vi "robot_state_machine1.vi"() -> ()   [LabVIEW 2015]
panel:
  out "angle error":dbl
  out "orientation theta desired":dbl
  out "start y":dbl
  out "start x 2":dbl=1.0
  out "x traveled 2":dbl
  out "y traveled 2":dbl
  out "avg 124":dbl
  out "avg 457":dbl
  out "psi dot 2":dbl
  out "distance traveled 2":dbl
  out "y dot 2":dbl
  out "x dot 2":dbl
  out "x position 2":dbl
  out "y position 2":dbl
  out "reset x y 2":dbl
  out "Tick Count(mSec) 2":u32 caption="Tick Count(mSec)"
  out "right":dbl
  out "left":dbl
  in  "x goal":dbl=10.0
  out "goal reached":bool=TRUE
  out "scale":dbl=1.0
  out "x/y":dbl
  out "stop switch":dbl=1.0
  in  "Encoder Reset":bool
  out "ENC.B_c.CNTR":i32
  out "ENC.B_b.CNTR":i32
  out "ENC.B_a.CNTR":i32
  out "ENC.A_c.CNTR":i32
  out "ENC.A_b.CNTR":i32
  out "ENC.A_a.CNTR":i32
  out "slope desired":dbl
  out "y desired":dbl
  in  "current angle":dbl
  in  "current y":dbl
  in  "stop motors":dbl
  in  "ypend 2":dbl
  in  "ypstart 2":dbl
  in  "yend straight":dbl=2.0
  out "d straight 2":dbl
  out "c straight 2":dbl
  out "b straight 2":dbl
  out "a straight 2":dbl
  out "slope straight 2":dbl
  in  "ypend turn":dbl
  in  "ypstart turn":dbl
  in  "yend turn":dbl=2.0
  in  "ystart turn":dbl=1.0
  out "d turn":dbl
  out "c turn":dbl
  out "b turn":dbl
  out "a turn":dbl
  out "slope turn":dbl
  out "a straight 1":dbl
  out "b straight 1":dbl
  out "c straight 1":dbl
  out "d straight 1":dbl
  in  "ystart":dbl=1.0
  in  "yend straight 1":dbl=2.0
  in  "ypstart straight 1":dbl
  in  "ypend straight 1":dbl
  in  "start x":dbl
  in  "dumping complete":bool
  in  "straight 2 end":dbl=10.0
  in  "turn end":dbl=7.0
  in  "straight 1 end":dbl=2.0
  in  "digging complete?":bool
  in  "current x":dbl
  in  "mining x":dbl=10.0
  in  "position good?":bool
  in  "mining location":dbl=1.0
  in  "case":dbl
  in  "state":dbl
  # "case 1 parameters\nstraight"
  # "state 0 start up parameters"
  # "case 1 start up parameters"
  # "state 2 dig control"
  # "case 0 start up parameters"
  # "state 4 dump control"
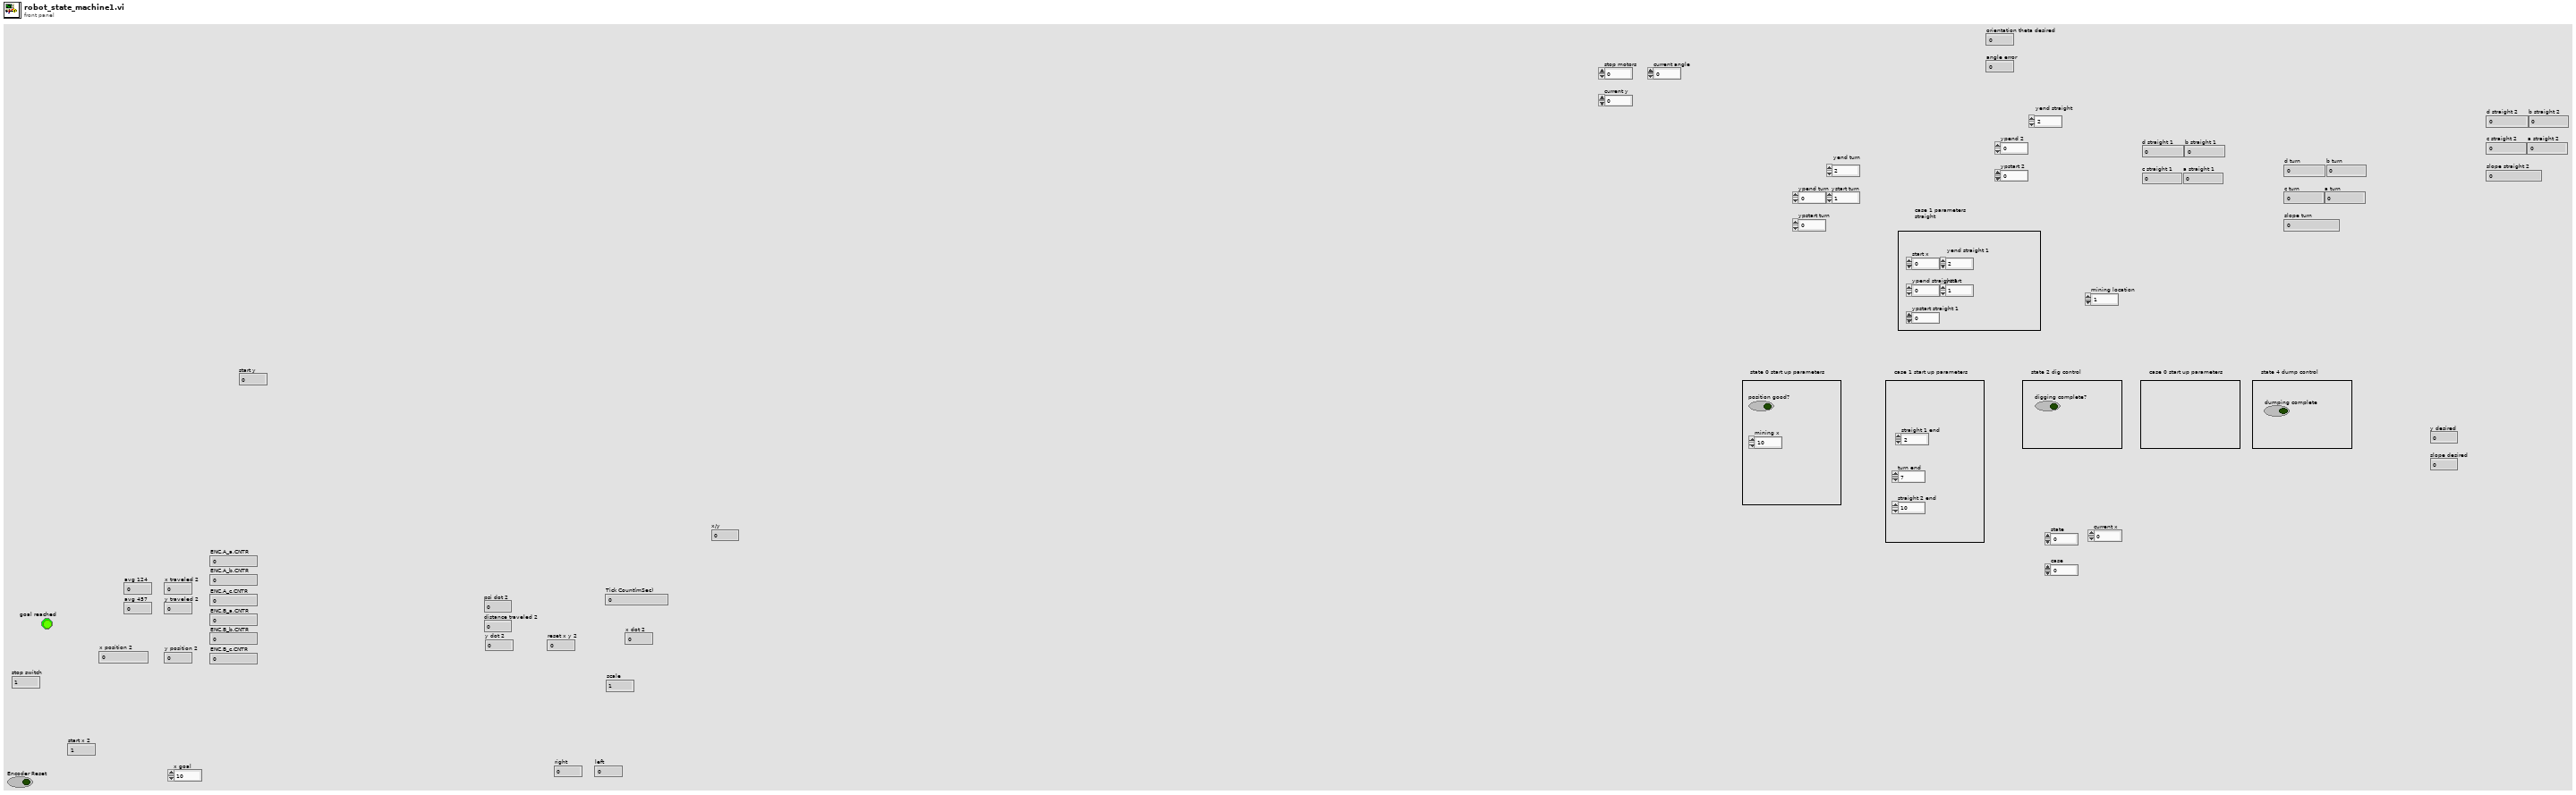
[diagram p1: front panel]
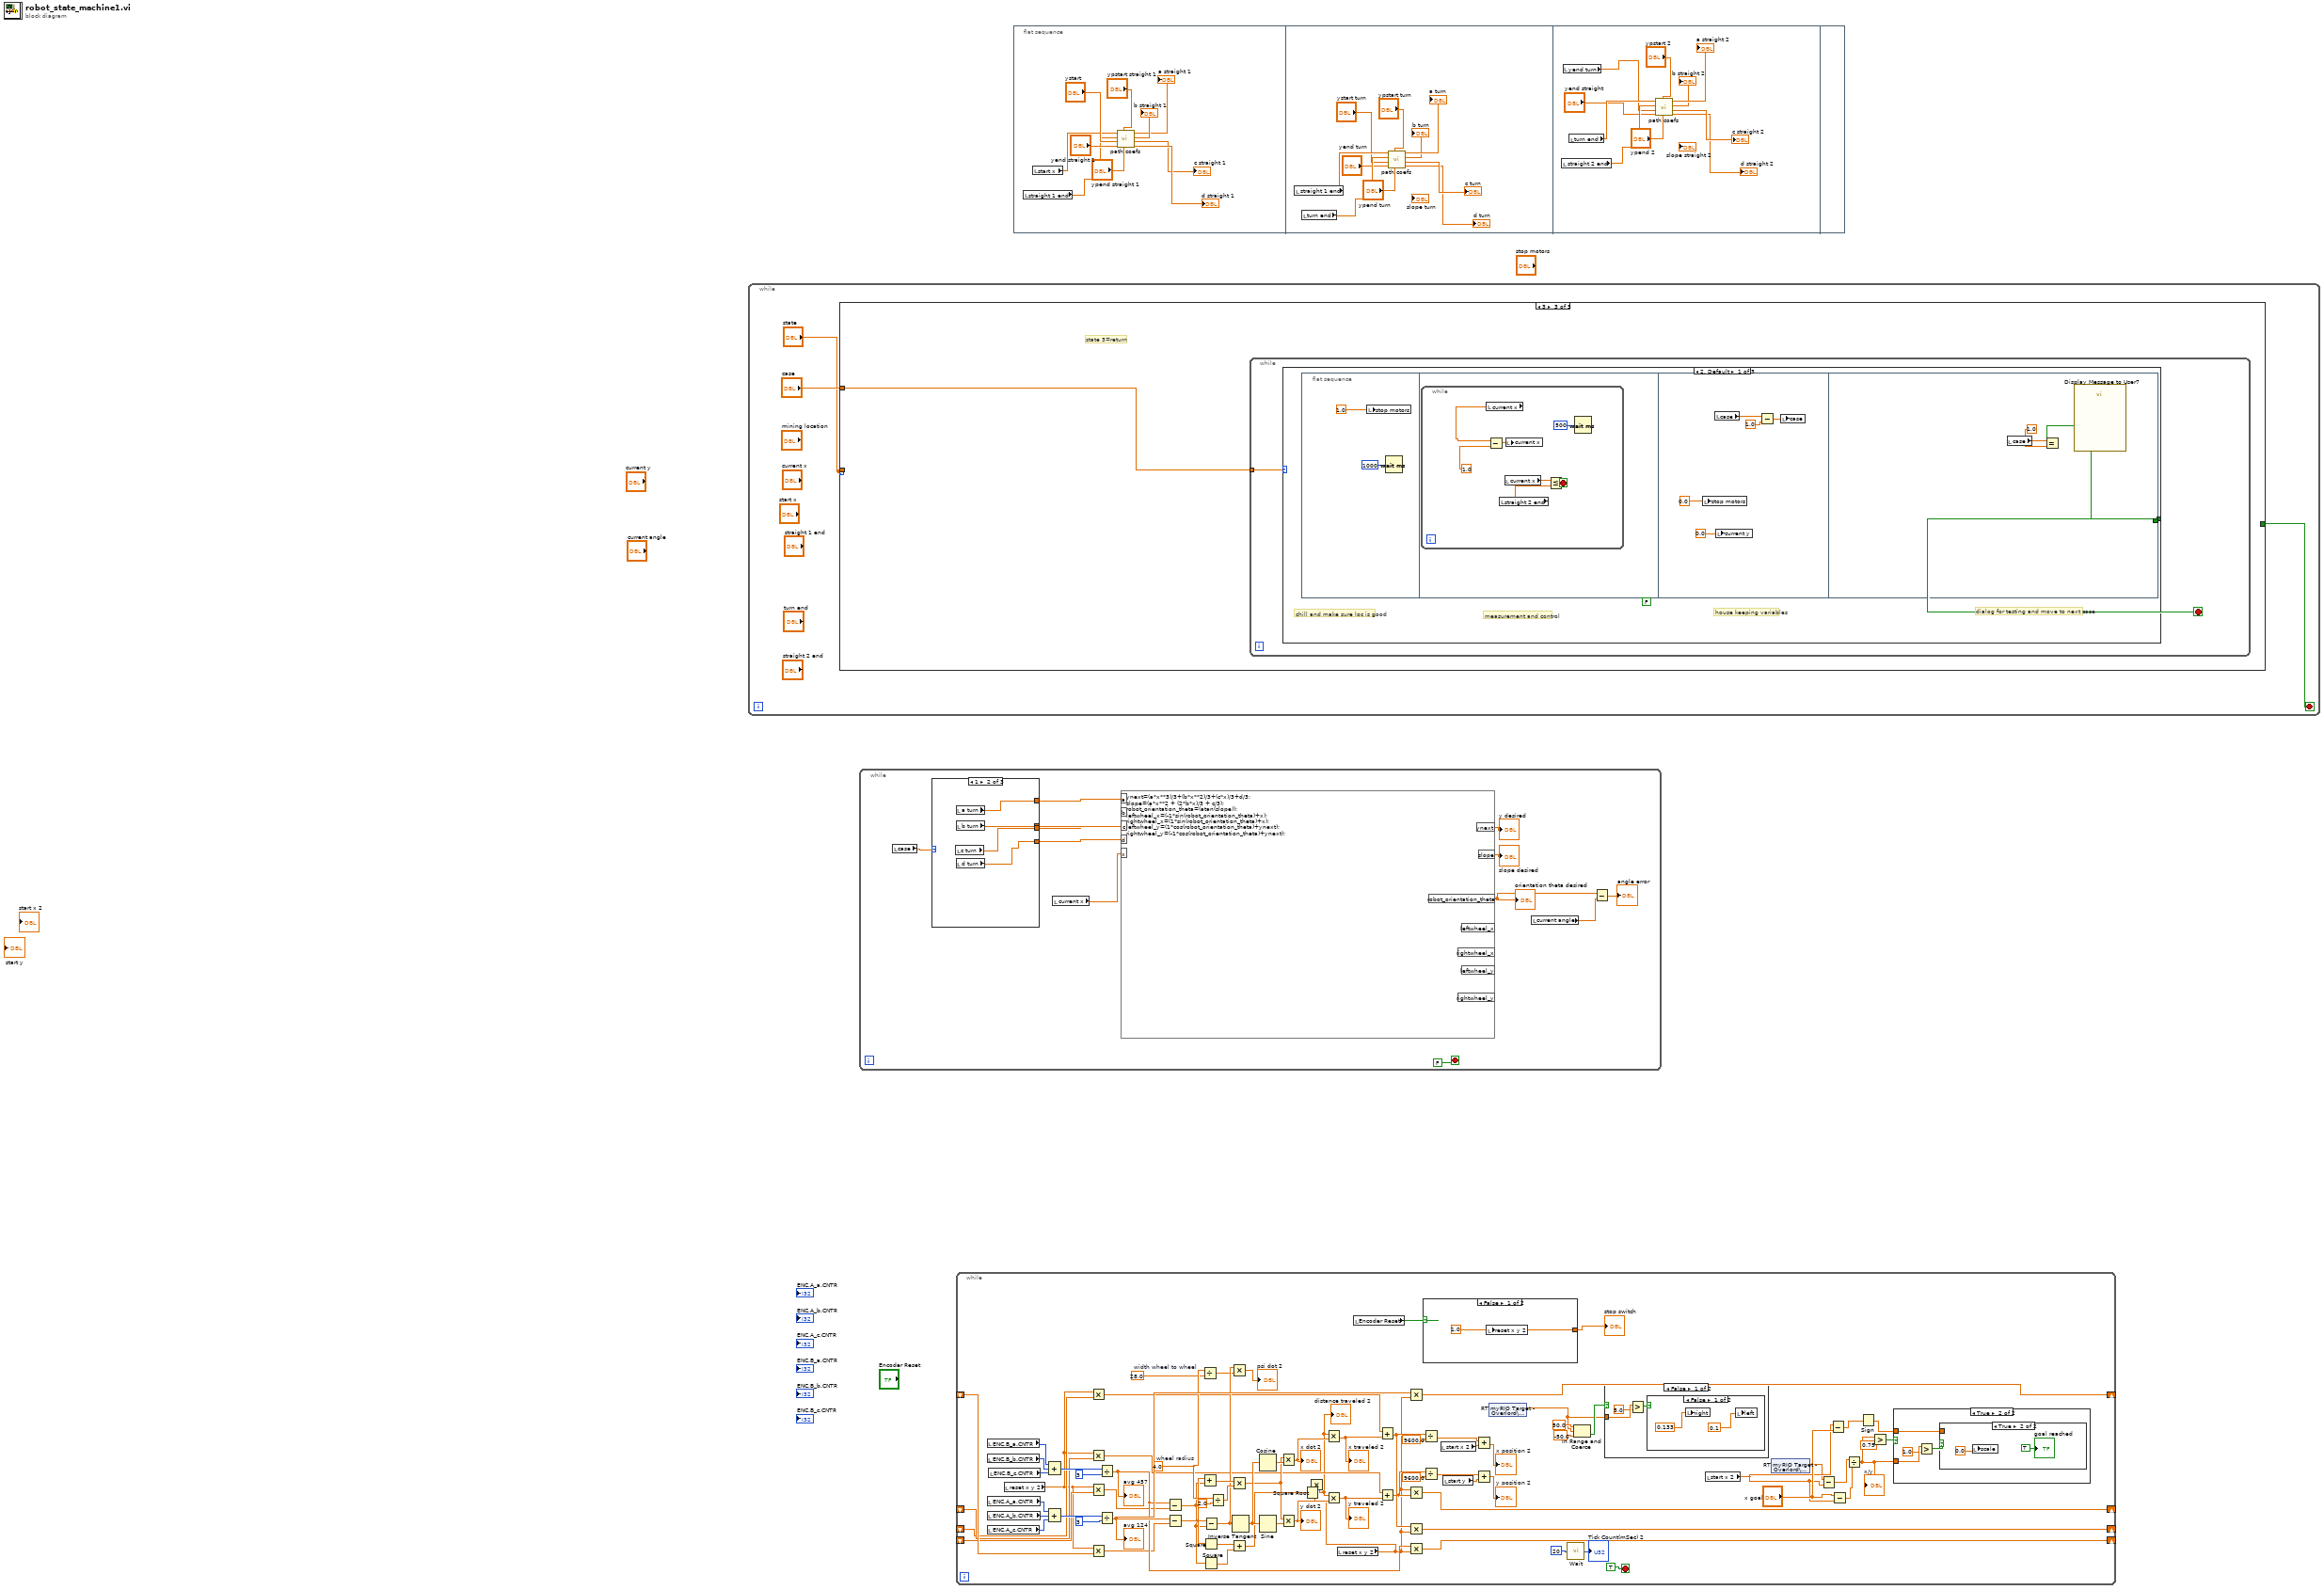
[diagram p0: block diagram]
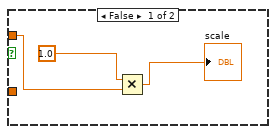
[diagram p2: hidden frame]
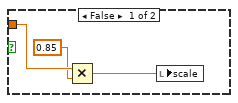
[diagram p3: hidden frame]
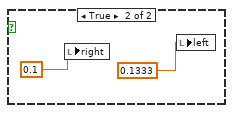
[diagram p4: hidden frame]
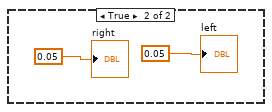
[diagram p5: hidden frame]
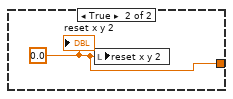
[diagram p6: hidden frame]
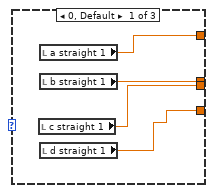
[diagram p7: hidden frame]
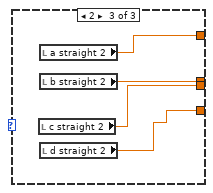
[diagram p8: hidden frame]
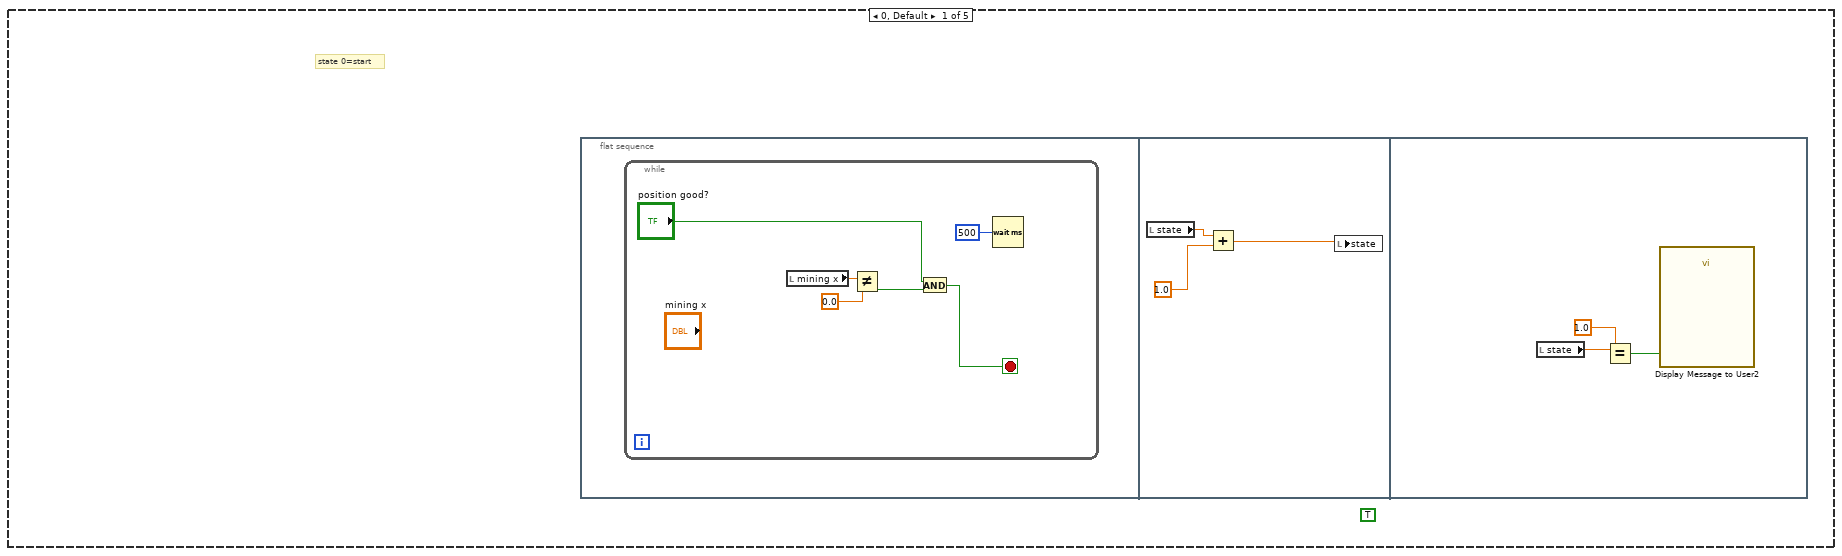
[diagram p9: hidden frame]
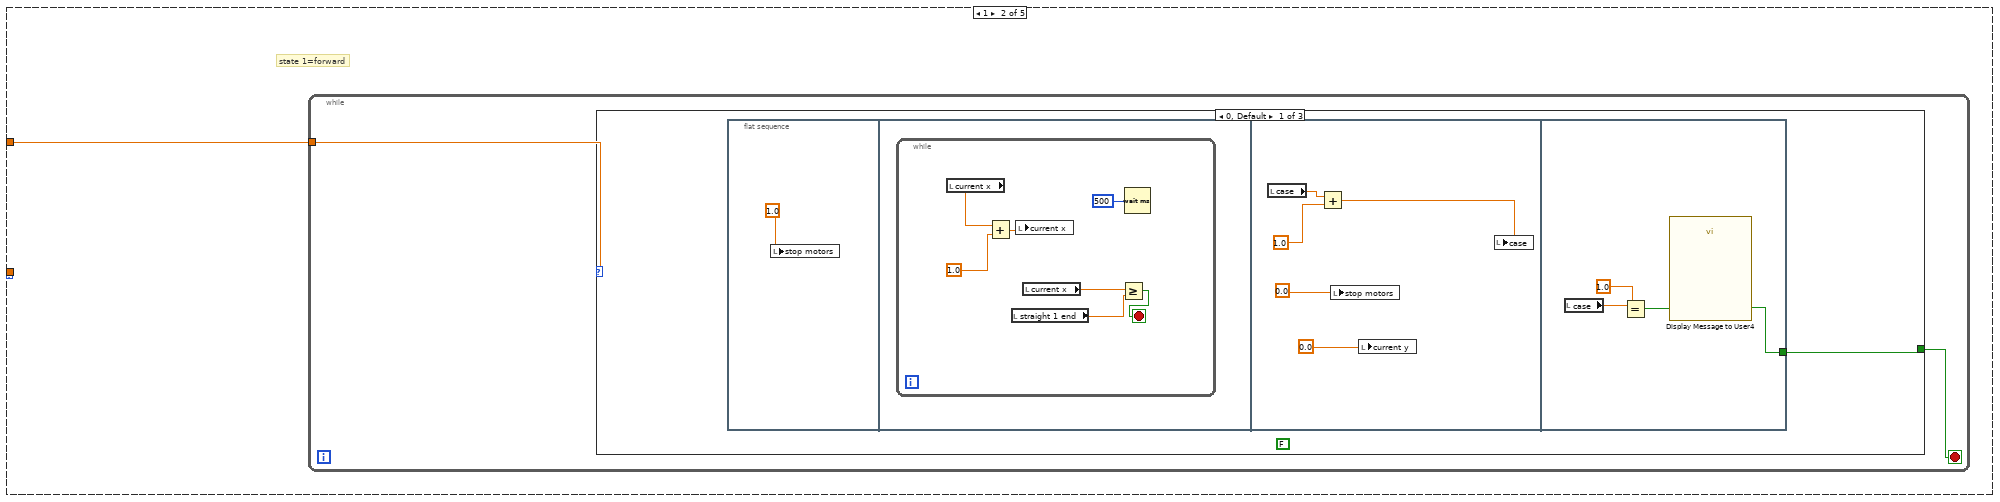
[diagram p10: hidden frame]
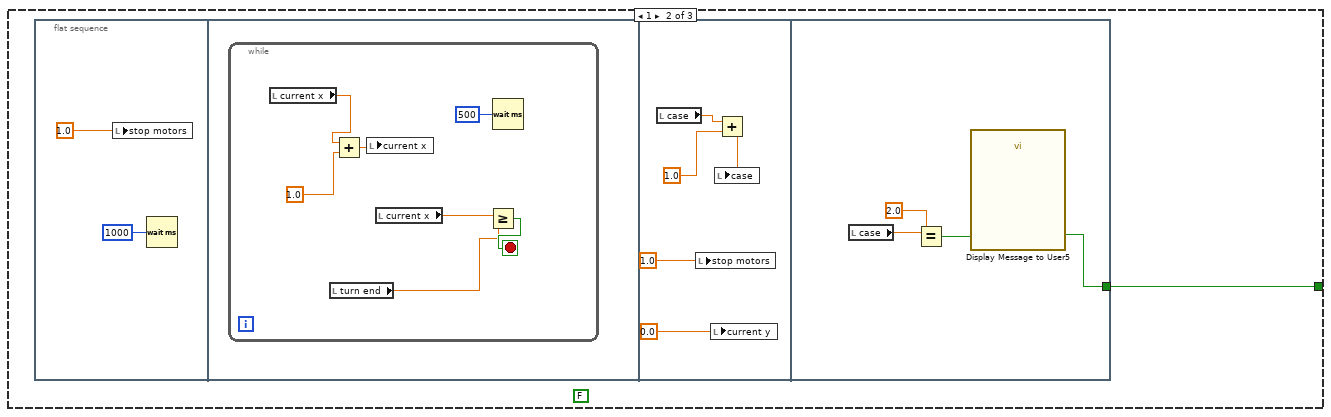
[diagram p11: hidden frame]
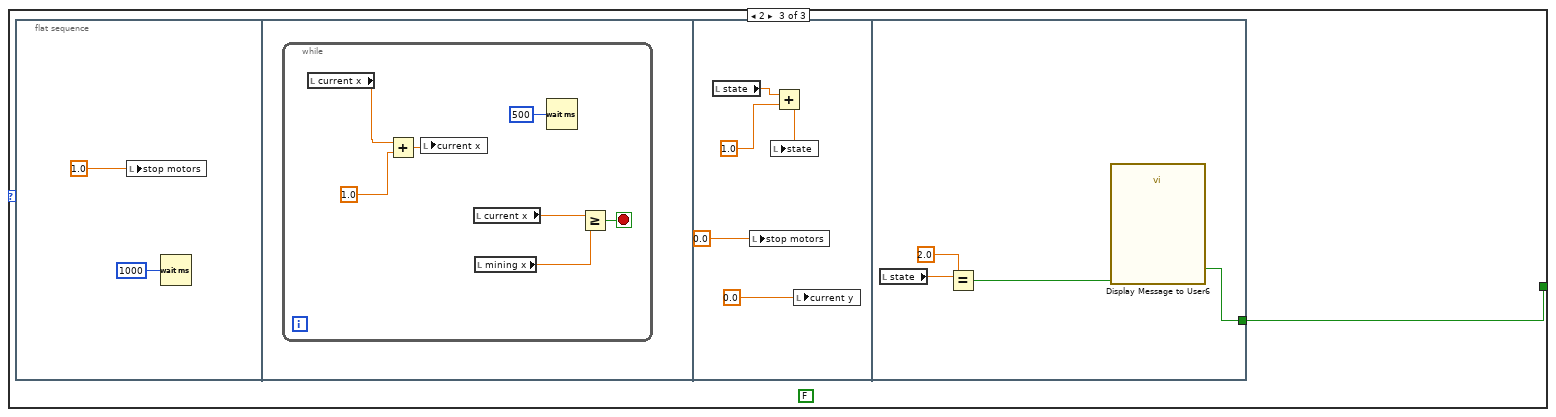
[diagram p12: hidden frame]
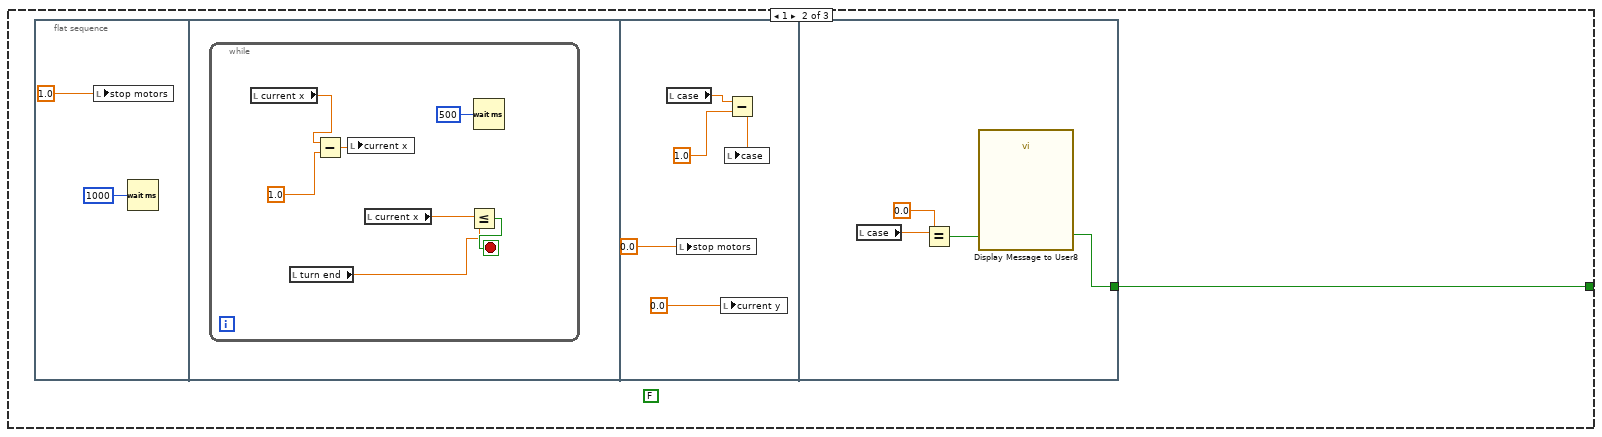
[diagram p13: hidden frame]
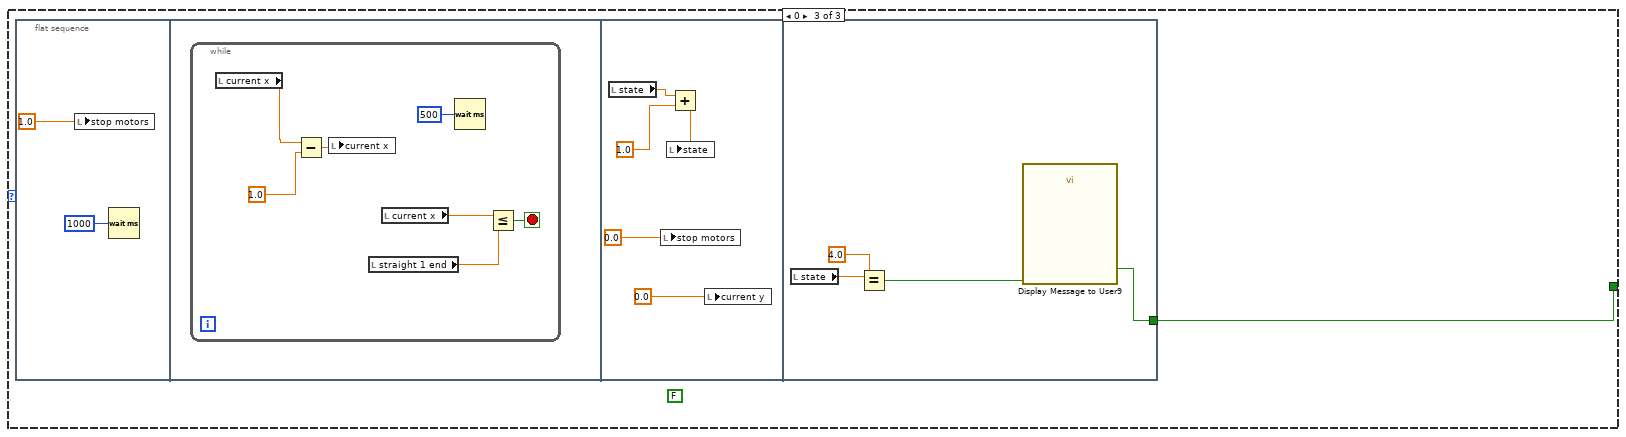
[diagram p14: hidden frame]
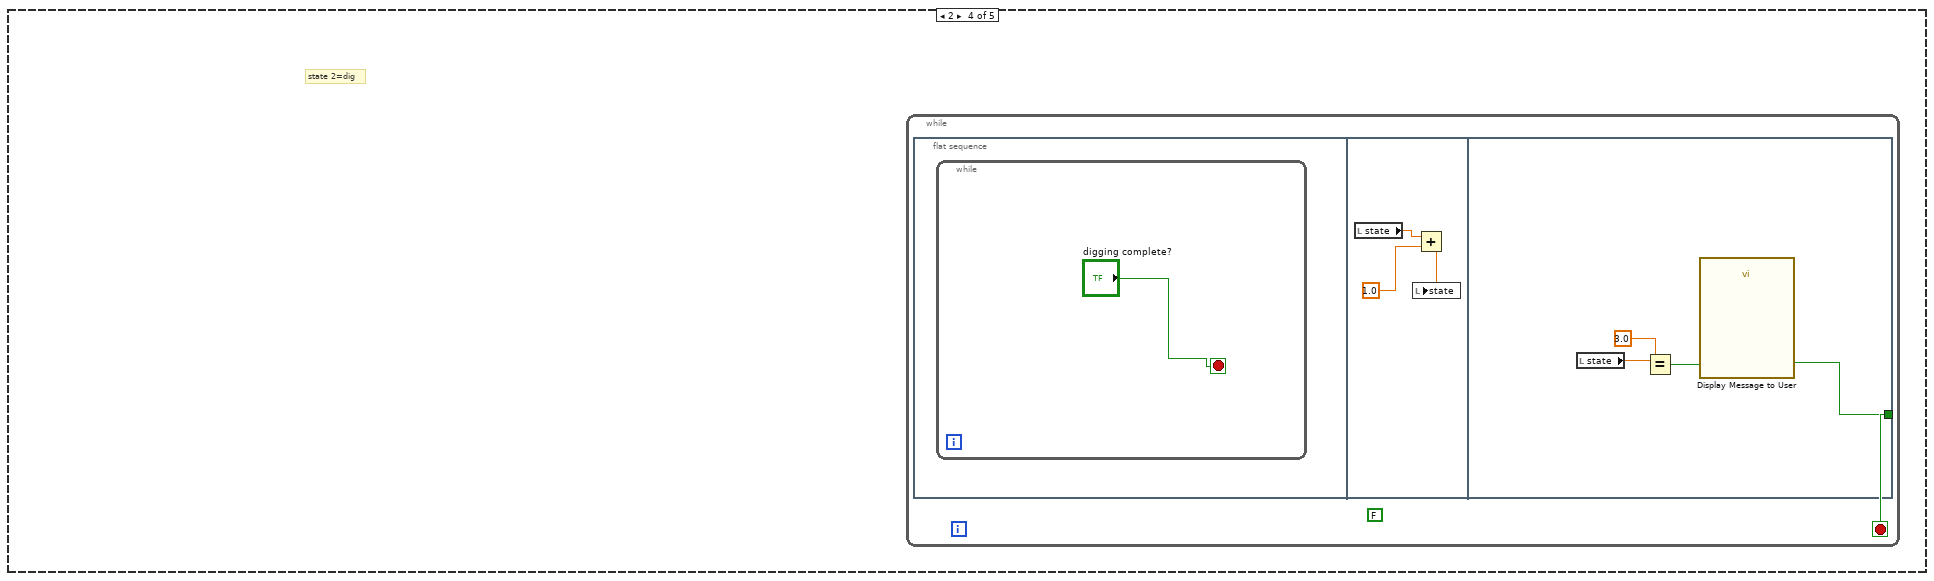
[diagram p15: hidden frame]
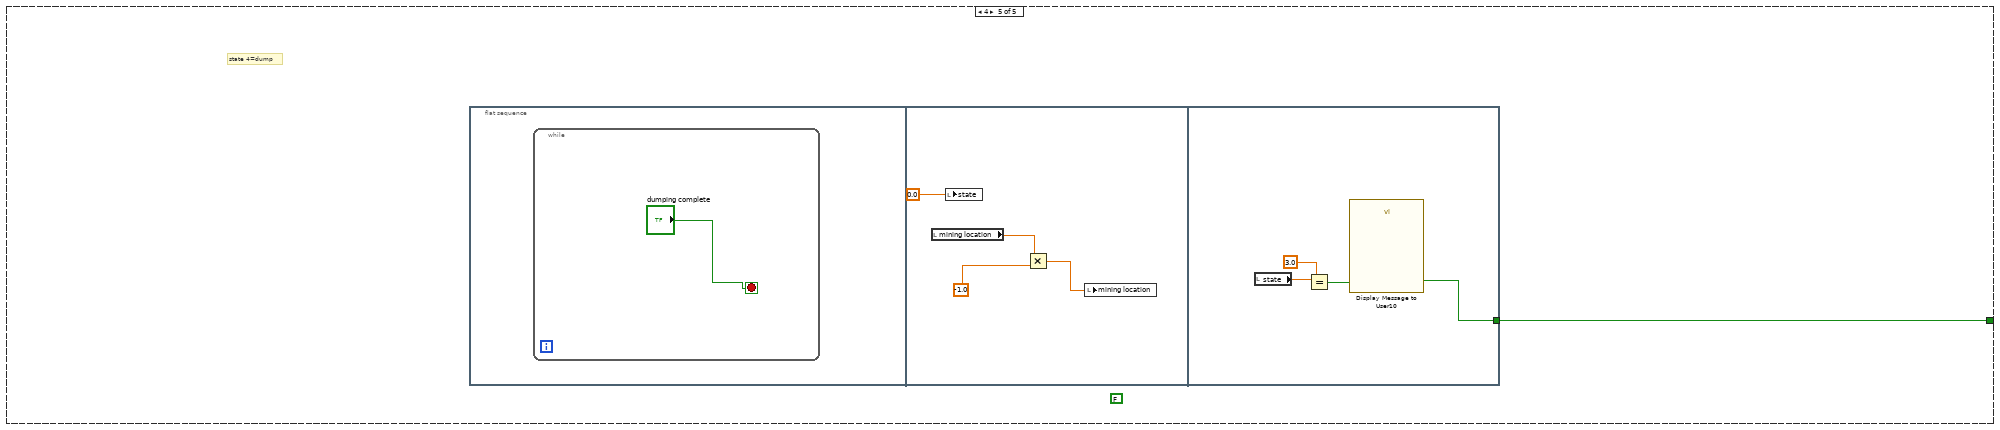
[diagram p16: hidden frame]
diagram:
  n1 = while {
    stop <- w3 stop-if-true
    n2 = case shown="3" "state" {
      tunnel: [_ _ _ _ w144] -> w3
      tunnel: "case" -> [_ w16 w75 _ _]
      tunnel: "state" -> [_ _ _ _ _]
      frame 0, Default {
        (unwired) TRUE
        # "state 0=start"
        n3 = flat-sequence {
          frame #0 {
            n4 = while {
              stop <- w4 stop-if-true
              n5 = local read "mining x"() -> (w9:dbl)
              n6 = Not Equal?(x=w9, y=0.0) -> (x != y?=w5:bool)
              n7 = And(x="position good?", y=w5) -> (x .and. y?=w4:bool)
              n8 = Wait (ms)(milliseconds to wait=u32 500) -> ()  [unwired: 1 out]
            }
          }
          frame #1 {
            n9 = local read "state"() -> (w10:dbl)
            n10 = Add(x=w10, y=1.0) -> (x+y=w12:dbl)
            n11 = local write "state"(w12) -> ()
          }
          frame #2 {
            n12 = local read "state"() -> (w15:dbl)
            n13 = Equal?(x=w15, y=1.0) -> (x = y?=w13:bool)
            n14 = call "Display Message to User2"("Enable"=w13) -> ()  [unwired: 9 in, 2 out]
          }
        }
      }
      frame 1 {
        # "state 1=forward"
        n15 = while {
          tunnel: w16 -> [w17]
          stop <- w18 stop-if-true
          n16 = case shown="0, Default" w17 {
            tunnel: [w19 w37 w56] -> w18
            frame 0, Default {
              (unwired) FALSE
              n17 = flat-sequence {
                tunnel: [w33] -> w19
                frame #0 {
                  n18 = local write "stop motors"(1.0) -> ()
                }
                frame #1 {
                  n19 = while {
                    stop <- w25 stop-if-true
                    n20 = local read "current x"() -> (w21:dbl)
                    n21 = Add(x=w21, y=1.0) -> (x+y=w26:dbl)
                    n22 = local read "straight 1 end"() -> (w22:dbl)
                    n23 = local write "current x"(w26) -> ()
                    n24 = local read "current x"() -> (w24:dbl)
                    n25 = Greater Or Equal?(x=w24, y=w22) -> (x >= y?=w25:bool)
                    n26 = Wait (ms)(milliseconds to wait=u32 500) -> ()  [unwired: 1 out]
                  }
                }
                frame #2 {
                  n27 = local read "case"() -> (w30:dbl)
                  n28 = Add(x=w30, y=1.0) -> (x+y=w32:dbl)
                  n29 = local write "stop motors"(0.0) -> ()
                  n30 = local write "current y"(0.0) -> ()
                  n31 = local write "case"(w32) -> ()
                }
                frame #3 {
                  n32 = local read "case"() -> (w36:dbl)
                  n33 = Equal?(x=w36, y=1.0) -> (x = y?=w34:bool)
                  n34 = call "Display Message to User4"("Enable"=w34) -> ("OK"=w33:bool)  [unwired: 9 in, 1 out]
                }
              }
            }
            frame 1 {
              (unwired) FALSE
              n35 = flat-sequence {
                tunnel: [w52] -> w37
                frame #0 {
                  n36 = local write "stop motors"(1.0) -> ()
                  n37 = Wait (ms)(milliseconds to wait=u32 1000) -> ()  [unwired: 1 out]
                }
                frame #1 {
                  n38 = while {
                    stop <- w44 stop-if-true
                    n39 = local read "current x"() -> (w41:dbl)
                    n40 = local read "turn end"() -> (w40:dbl)
                    n41 = Add(x=w41, y=1.0) -> (x+y=w45:dbl)
                    n42 = local write "current x"(w45) -> ()
                    n43 = local read "current x"() -> (w43:dbl)
                    n44 = Greater Or Equal?(x=w43, y=w40) -> (x >= y?=w44:bool)
                    n45 = Wait (ms)(milliseconds to wait=u32 500) -> ()  [unwired: 1 out]
                  }
                }
                frame #2 {
                  n46 = local read "case"() -> (w49:dbl)
                  n47 = local write "stop motors"(1.0) -> ()
                  n48 = local write "current y"(0.0) -> ()
                  n49 = Add(x=w49, y=1.0) -> (x+y=w51:dbl)
                  n50 = local write "case"(w51) -> ()
                }
                frame #3 {
                  n51 = local read "case"() -> (w55:dbl)
                  n52 = Equal?(x=w55, y=2.0) -> (x = y?=w53:bool)
                  n53 = call "Display Message to User5"("Enable"=w53) -> ("OK"=w52:bool)  [unwired: 9 in, 1 out]
                }
              }
            }
            frame 2 {
              (unwired) FALSE
              n54 = flat-sequence {
                tunnel: [w71] -> w56
                frame #0 {
                  n55 = local write "stop motors"(1.0) -> ()
                  n56 = Wait (ms)(milliseconds to wait=u32 1000) -> ()  [unwired: 1 out]
                }
                frame #1 {
                  n57 = while {
                    stop <- w63 stop-if-true
                    n58 = local read "current x"() -> (w60:dbl)
                    n59 = Add(x=w60, y=1.0) -> (x+y=w64:dbl)
                    n60 = local write "current x"(w64) -> ()
                    n61 = local read "current x"() -> (w62:dbl)
                    n62 = local read "mining x"() -> (w59:dbl)
                    n63 = Wait (ms)(milliseconds to wait=u32 500) -> ()  [unwired: 1 out]
                    n64 = Greater Or Equal?(x=w62, y=w59) -> (x >= y?=w63:bool)
                  }
                }
                frame #2 {
                  n65 = local read "state"() -> (w68:dbl)
                  n66 = local write "stop motors"(0.0) -> ()
                  n67 = Add(x=w68, y=1.0) -> (x+y=w70:dbl)
                  n68 = local write "state"(w70) -> ()
                  n69 = local write "current y"(0.0) -> ()
                }
                frame #3 {
                  n70 = local read "state"() -> (w74:dbl)
                  n71 = Equal?(x=w74, y=2.0) -> (x = y?=w72:bool)
                  n72 = call "Display Message to User6"("Enable"=w72) -> ("OK"=w71:bool)  [unwired: 9 in, 1 out]
                }
              }
            }
          }
        }
      }
      frame 3 {
        # "state 3=return"
        n73 = while {
          tunnel: w75 -> [w76]
          stop <- w77 stop-if-true
          n74 = case shown="2, Default" w76 {
            tunnel: [w78 w97 w116] -> w77
            frame 2, Default {
              (unwired) FALSE
              # "dialog for testing and move to next case"
              # "measurement and control"
              # "chill and make sure loc is good"
              # "house keeping variables"
              n75 = flat-sequence {
                tunnel: [w93] -> w78
                frame #0 {
                  n76 = local write "stop motors"(1.0) -> ()
                  n77 = Wait (ms)(milliseconds to wait=u32 1000) -> ()  [unwired: 1 out]
                }
                frame #1 {
                  n78 = while {
                    stop <- w85 stop-if-true
                    n79 = local read "current x"() -> (w82:dbl)
                    n80 = Subtract(x=w82, y=1.0) -> (x-y=w86:dbl)
                    n81 = local read "straight 2 end"() -> (w81:dbl)
                    n82 = local read "current x"() -> (w84:dbl)
                    n83 = local write "current x"(w86) -> ()
                    n84 = Less Or Equal?(x=w84, y=w81) -> (x <= y?=w85:bool)
                    n85 = Wait (ms)(milliseconds to wait=u32 500) -> ()  [unwired: 1 out]
                  }
                }
                frame #2 {
                  n86 = local write "stop motors"(0.0) -> ()
                  n87 = local read "case"() -> (w90:dbl)
                  n88 = local write "current y"(0.0) -> ()
                  n89 = Subtract(x=w90, y=1.0) -> (x-y=w92:dbl)
                  n90 = local write "case"(w92) -> ()
                }
                frame #3 {
                  n91 = local read "case"() -> (w96:dbl)
                  n92 = Equal?(x=w96, y=1.0) -> (x = y?=w94:bool)
                  n93 = call "Display Message to User7"("Enable"=w94) -> ("OK"=w93:bool)  [unwired: 9 in, 1 out]
                }
              }
            }
            frame 1 {
              (unwired) FALSE
              n94 = flat-sequence {
                tunnel: [w112] -> w97
                frame #0 {
                  n95 = local write "stop motors"(1.0) -> ()
                  n96 = Wait (ms)(milliseconds to wait=u32 1000) -> ()  [unwired: 1 out]
                }
                frame #1 {
                  n97 = while {
                    stop <- w104 stop-if-true
                    n98 = local read "current x"() -> (w101:dbl)
                    n99 = local read "turn end"() -> (w100:dbl)
                    n100 = Subtract(x=w101, y=1.0) -> (x-y=w105:dbl)
                    n101 = local write "current x"(w105) -> ()
                    n102 = local read "current x"() -> (w103:dbl)
                    n103 = Less Or Equal?(x=w103, y=w100) -> (x <= y?=w104:bool)
                    n104 = Wait (ms)(milliseconds to wait=u32 500) -> ()  [unwired: 1 out]
                  }
                }
                frame #2 {
                  n105 = local read "case"() -> (w110:dbl)
                  n106 = local write "stop motors"(0.0) -> ()
                  n107 = local write "current y"(0.0) -> ()
                  n108 = Subtract(x=w110, y=1.0) -> (x-y=w109:dbl)
                  n109 = local write "case"(w109) -> ()
                }
                frame #3 {
                  n110 = local read "case"() -> (w115:dbl)
                  n111 = Equal?(x=w115, y=0.0) -> (x = y?=w113:bool)
                  n112 = call "Display Message to User8"("Enable"=w113) -> ("OK"=w112:bool)  [unwired: 9 in, 1 out]
                }
              }
            }
            frame 0 {
              (unwired) FALSE
              n113 = flat-sequence {
                tunnel: [w131] -> w116
                frame #0 {
                  n114 = local write "stop motors"(1.0) -> ()
                  n115 = Wait (ms)(milliseconds to wait=u32 1000) -> ()  [unwired: 1 out]
                }
                frame #1 {
                  n116 = while {
                    stop <- w123 stop-if-true
                    n117 = local read "current x"() -> (w120:dbl)
                    n118 = Subtract(x=w120, y=1.0) -> (x-y=w124:dbl)
                    n119 = local write "current x"(w124) -> ()
                    n120 = local read "straight 1 end"() -> (w119:dbl)
                    n121 = local read "current x"() -> (w122:dbl)
                    n122 = Wait (ms)(milliseconds to wait=u32 500) -> ()  [unwired: 1 out]
                    n123 = Less Or Equal?(x=w122, y=w119) -> (x <= y?=w123:bool)
                  }
                }
                frame #2 {
                  n124 = local read "state"() -> (w128:dbl)
                  n125 = local write "stop motors"(0.0) -> ()
                  n126 = Add(x=w128, y=1.0) -> (x+y=w130:dbl)
                  n127 = local write "state"(w130) -> ()
                  n128 = local write "current y"(0.0) -> ()
                }
                frame #3 {
                  n129 = local read "state"() -> (w134:dbl)
                  n130 = Equal?(x=w134, y=4.0) -> (x = y?=w132:bool)
                  n131 = call "Display Message to User9"("Enable"=w132) -> ("OK"=w131:bool)  [unwired: 9 in, 1 out]
                }
              }
            }
          }
        }
      }
      frame 2 {
        # "state 2=dig"
        n132 = while {
          stop <- w135 stop-if-true
          (unwired) FALSE
          n133 = flat-sequence {
            tunnel: [w140] -> w135
            frame #0 {
              n134 = while {
                stop <- "digging complete?" stop-if-true
              }
            }
            frame #1 {
              n135 = local read "state"() -> (w138:dbl)
              n136 = Add(x=w138, y=1.0) -> (x+y=w137:dbl)
              n137 = local write "state"(w137) -> ()
            }
            frame #2 {
              n138 = local read "state"() -> (w143:dbl)
              n139 = Equal?(x=w143, y=3.0) -> (x = y?=w141:bool)
              n140 = call "Display Message to User"("Enable"=w141) -> ("OK"=w140:bool)  [unwired: 9 in, 1 out]
            }
          }
        }
      }
      frame 4 {
        (unwired) FALSE
        # "state 4=dump"
        n141 = flat-sequence {
          tunnel: [w150] -> w144
          frame #0 {
            n142 = while {
              stop <- "dumping complete" stop-if-true
            }
          }
          frame #1 {
            n143 = local read "mining location"() -> (w148:dbl)
            n144 = local write "state"(0.0) -> ()
            n145 = Multiply(x=w148, y=-1.0) -> (x*y=w146:dbl)
            n146 = local write "mining location"(w146) -> ()
          }
          frame #2 {
            n147 = local read "state"() -> (w153:dbl)
            n148 = Equal?(x=w153, y=3.0) -> (x = y?=w151:bool)
            n149 = call "Display Message to User10"("Enable"=w151) -> ("OK"=w150:bool)  [unwired: 9 in, 1 out]
          }
        }
      }
    }
  }
  n150 = while {
    stop <- FALSE stop-if-true
    n151 = local read "case"() -> (w160:dbl)
    n152 = case shown="1" w160 {
      tunnel: [w169 w173 w177] -> w164
      tunnel: [w168 w172 w176] -> w163
      tunnel: [w167 w171 w175] -> w162
      tunnel: [w166 w170 w174] -> w161
      frame 0, Default {
        n153 = local read "c straight 1"() -> (w167:dbl)
        n154 = local read "a straight 1"() -> (w169:dbl)
        n155 = local read "b straight 1"() -> (w168:dbl)
        n156 = local read "d straight 1"() -> (w166:dbl)
      }
      frame 1 {
        n157 = local read "c turn"() -> (w171:dbl)
        n158 = local read "a turn"() -> (w173:dbl)
        n159 = local read "b turn"() -> (w172:dbl)
        n160 = local read "d turn"() -> (w170:dbl)
      }
      frame 2 {
        n161 = local read "c straight 2"() -> (w175:dbl)
        n162 = local read "a straight 2"() -> (w177:dbl)
        n163 = local read "b straight 2"() -> (w176:dbl)
        n164 = local read "d straight 2"() -> (w174:dbl)
      }
    }
    n165 = local read "current x"() -> (w159:dbl)
    n166 = formula code="ynext=(a*x**3)/3+(b*x**2)/3+(c*x)/3+d/3;\nslope=(a*x**2 + (2*b*x)/3 + c/3);\nrobot_orientation_theta=(atan(slope));\nleftwheel_x=(-1*sin(robot_orientation_theta)+x);\nrightwheel_x=(1*sin(robot_orientation_theta)+x);\nleftwheel_y=(1*cos(robot_orientation_theta)+ynext);\nrightwheel_y=(-1*cos(robot_orientation_theta)+ynext);"("a"=w164, "b"=w163, "c"=w162, "d"=w161, "x"=w159) -> ("ynext"=→"y desired":dbl, "slope"=→"slope desired":dbl, "robot_orientation_theta"=w156:dbl)  [unwired: 4 out]
    "orientation theta desired" <- w156
    n167 = local read "current angle"() -> (w155:dbl)
    n168 = Subtract(x=w156, y=w155) -> (x-y=→"angle error":dbl)
  }
  n169 = while {
    shift-right: [w204] -> _
    shift-left: _ -> [w242]
    shift-right: [w201] -> _
    shift-left: _ -> [w241]
    shift-right: [w203] -> _
    shift-left: _ -> [w216]
    shift-right: [w202] -> _
    shift-left: _ -> [w215]
    stop <- TRUE stop-if-true
    w237 = 28.0  # width wheel to wheel
    w238 = 4.0  # wheel radius
    n170 = local read "ENC.B_a.CNTR"() -> (w247:i32)
    n171 = local read "ENC.B_b.CNTR"() -> (w246:i32)
    n172 = local read "ENC.A_a.CNTR"() -> (w250:i32)
    n173 = local read "ENC.A_b.CNTR"() -> (w249:i32)
    n174 = local read "ENC.A_c.CNTR"() -> (w248:i32)
    n175 = local read "ENC.B_c.CNTR"() -> (w245:i32)
    n176 = local read "reset x y 2"() -> (w200:dbl)
    n177 = Compound Arithmetic op=ADD(w247, w246, w245) -> (w253:i32)
    n178 = Compound Arithmetic op=ADD(w250, w249, w248) -> (w254:i32)
    n179 = Multiply(x=w200, y=w215) -> (x*y=w206:dbl)
    n180 = Multiply(x=w200, y=w216) -> (x*y=w207:dbl)
    n181 = Multiply(x=w200, y=w241) -> (x*y=w205:dbl)
    n182 = Multiply(x=w200, y=w242) -> (x*y=w208:dbl)
    n183 = Divide(x=w253, y=3) -> (x/y=w240:dbl)
    "avg 457" <- w240
    n184 = Divide(x=w254, y=3) -> (x/y=w243:dbl)
    "avg 124" <- w243
    n185 = Subtract(x=w240, y=w205) -> (x-y=w230:dbl)
    n186 = Subtract(x=w243, y=w208) -> (x-y=w231:dbl)
    n187 = Divide(x=w238, y=w237) -> (x/y=w233:dbl)
    n188 = Add(x=w231, y=w230) -> (x+y=w235:dbl)
    n189 = Square(x=w231) -> (x^2=w228:dbl)
    n190 = Square(x=w230) -> (x^2=w229:dbl)
    n191 = Subtract(x=w231, y=w230) -> (x-y=w234:dbl)
    n192 = Divide(x=w238, y=2.0) -> (x/y=w236:dbl)
    n193 = Multiply(x=w234, y=w233) -> (x*y=→"psi dot 2":dbl)
    n194 = Multiply(x=w235, y=w236) -> (x*y=w224:dbl)
    n195 = Add(x=w228, y=w229) -> (x+y=w227:dbl)
    n196 = Inverse Tangent(1:w234) -> (0:w232:dbl)
    n197 = Cosine(x=w232) -> (cos(x)=w225:dbl)
    n198 = Sine(x=w232) -> (sin(x)=w226:dbl)
    n199 = Multiply(x=w224, y=w225) -> (x*y=w222:dbl)
    "x dot 2" <- w222
    n200 = Multiply(x=w224, y=w226) -> (x*y=w223:dbl)
    "y dot 2" <- w223
    n201 = Square Root(x=w227) -> (sqrt(x)=w221:dbl)
    n202 = local read "reset x y 2"() -> (w198:dbl)
    n203 = Multiply(x=w221, y=w198) -> (x*y=w199:dbl)
    "distance traveled 2" <- w199
    n204 = Multiply(x=w199, y=w222) -> (x*y=w220:dbl)
    "x traveled 2" <- w220
    n205 = Multiply(x=w199, y=w223) -> (x*y=w219:dbl)
    "y traveled 2" <- w219
    n206 = local read "Encoder Reset"() -> (w197:bool)
    n207 = Add(x=w206, y=w220) -> (x+y=w218:dbl)
    n208 = Add(x=w207, y=w219) -> (x+y=w210:dbl)
    n209 = Multiply(x=w243, y=w198) -> (x*y=w204:dbl)
    n210 = Multiply(x=w198, y=w210) -> (x*y=w203:dbl)
    n211 = Multiply(x=w218, y=w198) -> (x*y=w202:dbl)
    n212 = Multiply(x=w240, y=w198) -> (x*y=w201:dbl)
    n213 = Divide(x=w218, y=9600.0) -> (x/y=w213:dbl)
    n214 = Divide(x=w210, y=9600.0) -> (x/y=w214:dbl)
    n215 = case shown="False" w197 {
      tunnel: [w277 w278] -> w178
      frame False {
        w277 = 1.0
        n216 = local write "reset x y 2"(w277) -> ()
      }
      frame True {
        w278 = 0.0
        n217 = local write "reset x y 2"(w278) -> ()
        "reset x y 2" <- w278
      }
    }
    "stop switch" <- w178
    n218 = local read "start x 2"() -> (w211:dbl)
    n219 = local read "start y"() -> (w212:dbl)
    n220 = Add(x=w213, y=w211) -> (x+y=→"x position 2":dbl)
    n221 = Add(x=w214, y=w212) -> (x+y=→"y position 2":dbl)
    n222 = shared-variable "RT myRIO Target - Overlord\\Localization_Variables_r0.lvlib\\loc_x"() -> (w180:dbl)  [unwired: 1 in, 1 out]
    n223 = call "Wait"("Count(mSec)"=u32 20) -> ("Tick Count(mSec)"=→"Tick Count(mSec) 2":u32)
    n224 = In Range and Coerce(upper limit=50.0, x=w180, lower limit=-50.0) -> (In Range?=w191:bool)  [unwired: 1 out]
    n225 = case shown="False" w191 {
      tunnel: w180 -> [w270 _]
      frame False {
        n226 = Greater?(x=w270, y=5.0) -> (0:w268:bool)
        n227 = case shown="False" w268 {
          frame False {
            n228 = local write "right"(0.133) -> ()
            n229 = local write "left"(0.1) -> ()
          }
          frame True {
            n230 = local write "right"(0.1) -> ()
            n231 = local write "left"(0.1333) -> ()
          }
        }
      }
      frame True {
        "right" <- 0.05
        "left" <- 0.05
      }
    }
    n232 = local read "start x 2"() -> (w182:dbl)
    n233 = shared-variable "RT myRIO Target - Overlord\\Localization_Variables_r0.lvlib\\loc_x"() -> (w179:dbl)  [unwired: 1 in, 1 out]
    n234 = Subtract(x=w179, y=w182) -> (x-y=w187:dbl)
    n235 = Subtract(x=w182, y="x goal") -> (x-y=w184:dbl)
    n236 = Subtract(x="x goal", y=w182) -> (x-y=w186:dbl)
    n237 = Divide(x=w187, y=w186) -> (x/y=w188:dbl)
    "x/y" <- w188
    n238 = Sign(1:w184) -> (0:w183:dbl)
    n239 = Greater?(x=w188, y=0.75) -> (0:w189:bool)
    n240 = case shown="True" w189 {
      tunnel: w188 -> [_ w262]
      tunnel: w183 -> [w257 w259]
      frame False {
        n241 = Multiply(x=1.0, y=w257) -> (x*y=→"scale":dbl)
      }
      frame True {
        n242 = Greater?(x=w262, y=1.0) -> (0:w260:bool)
        n243 = case shown="True" w260 {
          tunnel: w259 -> [w265 _]
          frame False {
            n244 = Multiply(x=w265, y=0.85) -> (x*y=w263:dbl)
            n245 = local write "scale"(w263) -> ()
          }
          frame True {
            n246 = local write "scale"(0.0) -> ()
            "goal reached" <- TRUE
          }
        }
      }
    }
  }
  n247 = flat-sequence {
    frame #0 {
      n248 = local read "straight 1 end"() -> (w279:dbl)
      n249 = local read "start x"() -> (w280:dbl)
      n250 = call "path coefs.vi"("ypend"="ypend straight 1", "ypstart"="ypstart straight 1", "yend"="yend straight 1", "ystart"="ystart", "xend"=w279, "xstart"=w280) -> ("d"=→"d straight 1":dbl, "c"=→"c straight 1":dbl, "b"=→"b straight 1":dbl, "a"=→"a straight 1":dbl)  [unwired: 2 in]
    }
    frame #1 {
      n251 = local read "straight 1 end"() -> (w297:dbl)
      n252 = local read "turn end"() -> (w298:dbl)
      n253 = call "path coefs.vi"("ypend"="ypend turn", "ypstart"="ypstart turn", "yend"="yend turn", "ystart"="ystart turn", "xend"=w298, "xstart"=w297) -> ("d"=→"d turn":dbl, "c"=→"c turn":dbl, "b"=→"b turn":dbl, "a"=→"a turn":dbl)  [unwired: 2 in]
    }
    frame #2 {
      n254 = local read "straight 2 end"() -> (w308:dbl)
      n255 = local read "yend turn"() -> (w299:dbl)
      n256 = local read "turn end"() -> (w307:dbl)
      n257 = call "path coefs.vi"("ypend"="ypend 2", "ypstart"="ypstart 2", "yend"="yend straight", "ystart"=w299, "xend"=w308, "xstart"=w307) -> ("d"=→"d straight 2":dbl, "c"=→"c straight 2":dbl, "b"=→"b straight 2":dbl, "a"=→"a straight 2":dbl)  [unwired: 2 in]
    }
    frame #3 {
    }
  }
